vi "CRYConvert Unicode to Multibyte.vi"(8 "error in":errorcluster, 9 "Code Page":u32(ring) items=["System default"=0, "Latin-1"=1252, "Japanese"=932, "Korean"=949, "Chinese simplified"=936, "Chinese traditional"=950, "Central Europe"=1250, "Cyrillic"=1251, "Greek"=1253, "Turkish"=1254, "Hebrew"=1255, "Arabic"=1256, "Baltic"=1257, "Thai"=874, "Vietnamese"=783, "UTF8"=65001, "UTF-7"=65000], 10 "Big Endian?":bool, 11 "Unicode String":string) -> (0 "error out":errorcluster, 3 "Multibyte string":string)   [LabVIEW 2013]
uses:
  Kernel32.DLL
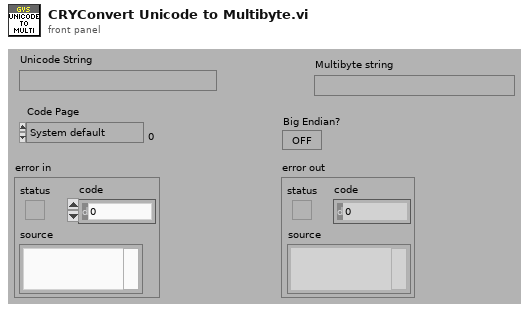
[diagram p1: front panel]
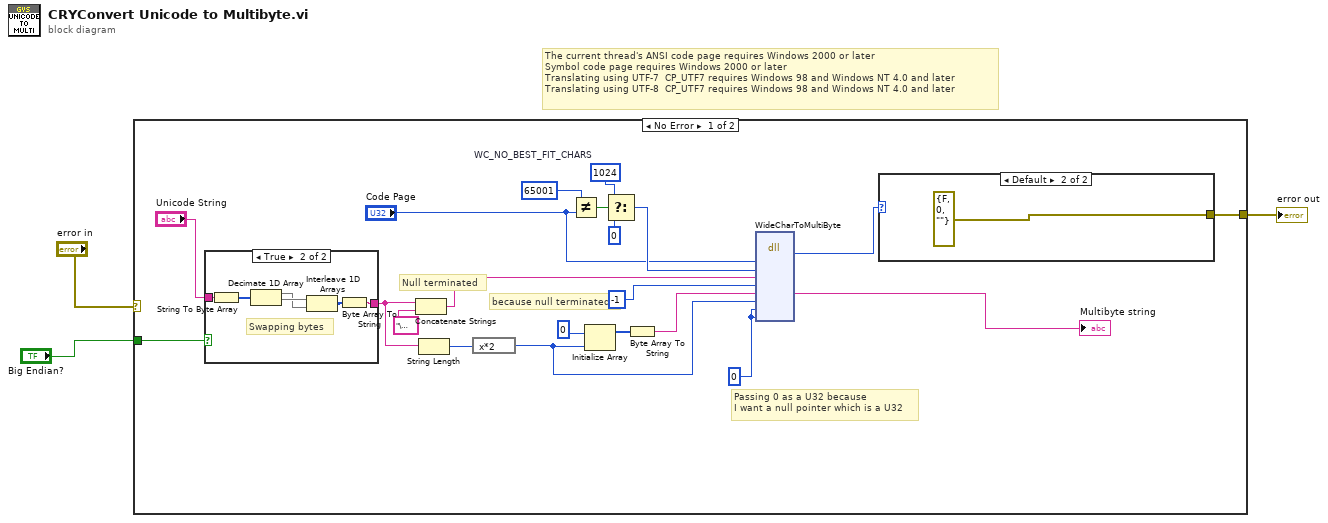
[diagram p0: block diagram]
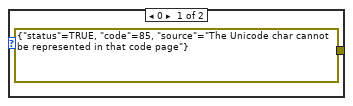
[diagram p3: hidden frame]
diagram:
  # "The current thread's ANSI code page requires Windows 2000 or later\nSymbol code page requires Windows 2000 or later\nTranslating using UTF-7  CP_UTF7 requires Windows 98 and Windows NT 4.0 and later\nTranslating using UTF-8  CP_UTF7 requires Windows 98 and Windows NT 4.0 and later"
  n1 = case shown="No Error" "error in" {
    selector: "error in" -> [_ w34]
    tunnel: [w7 w34] -> w3
    tunnel: "Big Endian?" -> [w6 _]
    frame No Error {
      w9 = u32 0 ("usedefault")
      w22 = u32 1024  # WC_NO_BEST_FIT_CHARS
      # "Passing 0 as a U32 because\nI want a null pointer which is a U32"
      # "because null terminated"
      # "Null terminated"
      n2 = case shown="True" w6 {
        tunnel: "Unicode String" -> [w25 w27]
        tunnel: [w25 w26] -> w12
        frame False {
        }
        frame True {
          # "Swapping bytes"
          n3 = String To Byte Array(string=w27) -> (unsigned byte array=w28:u8[])
          n4 = Decimate 1D Array(w28) -> (w30:u8[], w31:u8[])
          n5 = Interleave 1D Arrays(w31, w30) -> (w29:u8[])
          n6 = Byte Array To String(unsigned byte array=w29) -> (string=w26:string)
        }
      }
      n7 = Concatenate Strings(w12, "\u0000" ("chaîne")) -> (w16:string)
      n8 = String Length(string=w12) -> (length=w14:i32)
      n9 = expression code="x*2"(w14) -> (w11:i32)
      n10 = Not Equal?(x=u32 65001, y="Code Page") -> (x != y?=w23:bool)
      n11 = Initialize Array(u8 0, w11) -> (w19:u8[])
      n12 = Select(t=w22, s=w23, f=u32 0) -> (s? t:f=w10:u32)
      n13 = Byte Array To String(unsigned byte array=w19) -> (string=w18:string)
      n14 = dll-call lib="Kernel32.DLL" fn="WideCharToMultiByte"("Codepage"="Code Page", "dwFlags"=w10, "widestring"=w16, "nbchar"=-1, "buffernewstring"=w18, "buffersize"=w11, "defaultchar"=w9, "usedefault"=w9) -> (w8:i32, "buffernewstring"=→"Multibyte string":string)  [unwired: 10 in, 2 out]
      n15 = case shown="Default" w8 {
        tunnel: [errorcluster {"status"=TRUE, "code"=85, "source"="The Unicode char cannot be represented in that code page"} ("error out") errorcluster {"status"=FALSE, "code"=0, "source"=""} ("error out")] -> w7
        frame 0 {
        }
        frame Default {
        }
      }
    }
    frame Error {
    }
  }
  "error out" <- w3
